vi "Get Name from Class ID.vi"(1 "Class ID":u32) -> (0 "Get Class Name From Class ID":string)   [LabVIEW 2018]
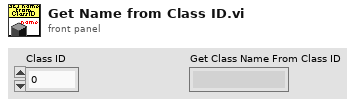
[diagram p1: front panel]
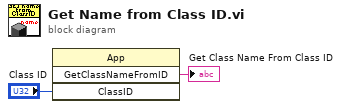
[diagram p0: block diagram]
diagram:
  n1 = invoke class="App" method="GetClassNameFromID"("ClassID"="Class ID") -> ("GetClassNameFromID"=→"Get Class Name From Class ID":string)  [unwired: 3 in, 3 out]
